vi "LEP_RV_MemoryMap_TCP.vi"(8 "error in (no error)":errorcluster, 11 "Target":string="Build Spec Name") -> (0 "error out":errorcluster)   [LabVIEW 2011]
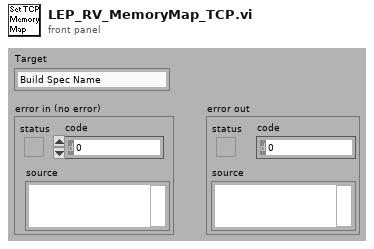
[diagram p1: front panel]
types:
  T1 = enum32{"Unused", "OPT_LMISC", "OPT_CMISC", "OPT_AMISC", "OPT_CINCL", "OPT_AINCL", "OPT_CDEF", "OPT_ADEF", "OPT_CUNDEF", "OPT_AUNDEF", "OPT_COPTIMIZE", "OPT_CODEGEN", "OPT_MEMRANGES", "OPT_ASNMEMRANGES"}
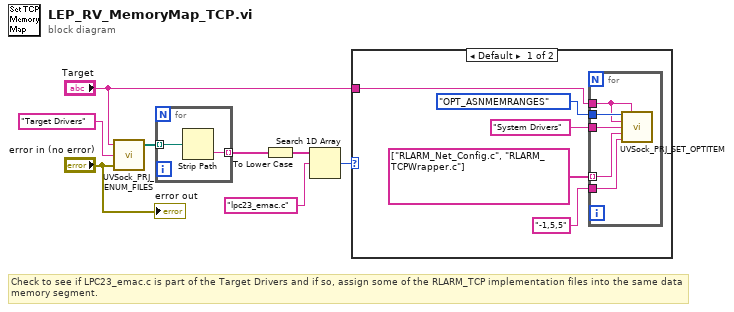
[diagram p0: block diagram]
diagram:
  # "Check to see if LPC23_emac.c is part of the Target Drivers and if so, assign some of the RLARM_TCP implementation files into the same data memory segment."
  n1 = call "UVSock_PRJ_ENUM_FILES.vi"("error in (no error)"="error in (no error)", "Group"="Target Drivers", "Target"="Target") -> ("Files"=w7:path[])  [unwired: 2 out]
  n2 = for {
    tunnel: w7 -> [w10] mode=indexing
    tunnel: [w9] -> w6 mode=indexing
    n3 = Strip Path(path=w10) -> (name=w9:string)  [unwired: 1 out]
  }
  n4 = To Lower Case(string=w6) -> (all lower case string=w5:string[])
  n5 = Search 1D Array(1D array=w5, element="lpc23_emac.c") -> (index of element=w3:i32)  [unwired: 1 out]
  n6 = case shown="Default" w3 {
    tunnel: "Target" -> [w14 _]
    frame Default {
      n7 = for {
        tunnel: T1."OPT_ASNMEMRANGES" ("Option In") -> [w20]
        tunnel: w14 -> [w19]
        tunnel: "System Drivers" ("Group Name In") -> [w18]
        tunnel: string[] ["RLARM_Net_Config.c", "RLARM_TCPWrapper.c"] -> [w17] mode=indexing
        tunnel: "-1,5,5" -> [w16]
        n8 = call "UVSock_PRJ_SET_OPTITEM.vi"("Option In"=w20, "Target"=w19, "Target Name In"=w19, "Group Name In"=w18, "File Name In"=w17, "Item In"=w16) -> ()  [unwired: 1 in, 9 out]
      }
    }
    frame -1 {
    }
  }
  "error out" <- "error in (no error)"
